vi "KDTHN_Main.vi"() -> ()   [LabVIEW 2018]
doc: "This VIs aim to control both PicoScope 2204A and Arduino UNO3 with ADS9850BRS to gen sinunoid signal with different frequencies\n\nProgrammer: myselfHungNN\n0968354050\nhungtd@mta.edu.vn"
uses:
  LVDrivers_Instruments/uno3/uno3.lvlib
  <vilib>/ErrorRing/Error Ring.xnode
  type defs/TimeBase Cluster.ctl
  type defs/Trigger Cluster.ctl
  type defs/Ranges.ctl
  type defs/Channel Settings.ctl
  type defs/Pico Cluster.ctl
  type defs/Channel Selection.ctl
  LVDrivers_Instruments/picoscope2000a/picoscope2000.lvlib
  type defs/App Cluster.ctl
  type defs/AmplifierTypes.ctl
  type defs/OpAmp Amplifiers.ctl
  <vilib>/Instr/_visa.llb/VISA Configure Serial Port (Instr).vi
panel:
  out "Time left":string
  out "Ngµy & Giê":string
  in  "Test?":bool
  in  "capture":bool caption="L­u mµn h×nh"
  in  "D÷ liÖu  ®o":string[][](table)
  in  "Trans":bool
  in  "OpAmp":bool
  in  "Opamp Type":T1=enum."NO Amplifier" caption="OpAmp"
  in  "Play Button":bool
  in  "Offset":dbl
  in  "Range 2":T2=enum."5 V"
  in  "Coupling":i16(ring)=1 items=["AC", "DC"]
  in  "Enabled":bool=TRUE
  in  "Offset":dbl
  in  "Range":T2=enum."5 V"
  in  "Coupling":i16(ring)=1 items=["AC", "DC"]
  in  "Enabled":bool=TRUE
  in  "Tab Control":enum32{"D¹ng sãng tÝn hiÖu", "Phæ tÝn hiÖu"}(tab)
  out "Time":waveform(dbl)[](graph)
  out "Freq":waveform(dbl)[](graph)
  in  "Disconnect":bool
  in  "Connect":bool
  out "sent":string
  out "number":u8
  out "UNO Rep":string
  in  "# Samples":i32=6000
  in  "Timebase":i16=3
  in  "Direction":i16(ring) items=["Rising", "Falling"]
  in  "Source":i16(ring)=5 items=["Ch A", "Ch B", "Ch C", "Ch D", "Ext", "None"]
  in  "Threshold mV":i16
  out "Actual Sampling Time ns":dbl caption="Actual Sampling Time [ns]"
  out "stop":bool
  in  "Cæng kÕt nèi":refnum<visa-resource-name>="COM4"
  in  "Test Error":bool
  in  "Amplifier Type":T3 caption="Trans Type"
  in  "Amplitude(Volts)":u8(knob)=1 max=10 step=1 scale=0.0..10.0
  in  "Frequency(Hz)":dbl(knob) min=0.0 max=1500000.0 scale=500.0..1500000.0
  in  "Quit Button":bool
  # "M¸Y PH¸T TÝN HIÖU"
  # "M¸Y HIÖN SãNG"
  # "Chan A"
  # "Chan B"
  # "Trigger"
  # "TimeDiv"
  # "khoa v« tuyÕn ®iÖn tö\nBé m«n C¬ së kü thuËt v« tuyÕn"
  # "AMPL"
  # "FREQ"
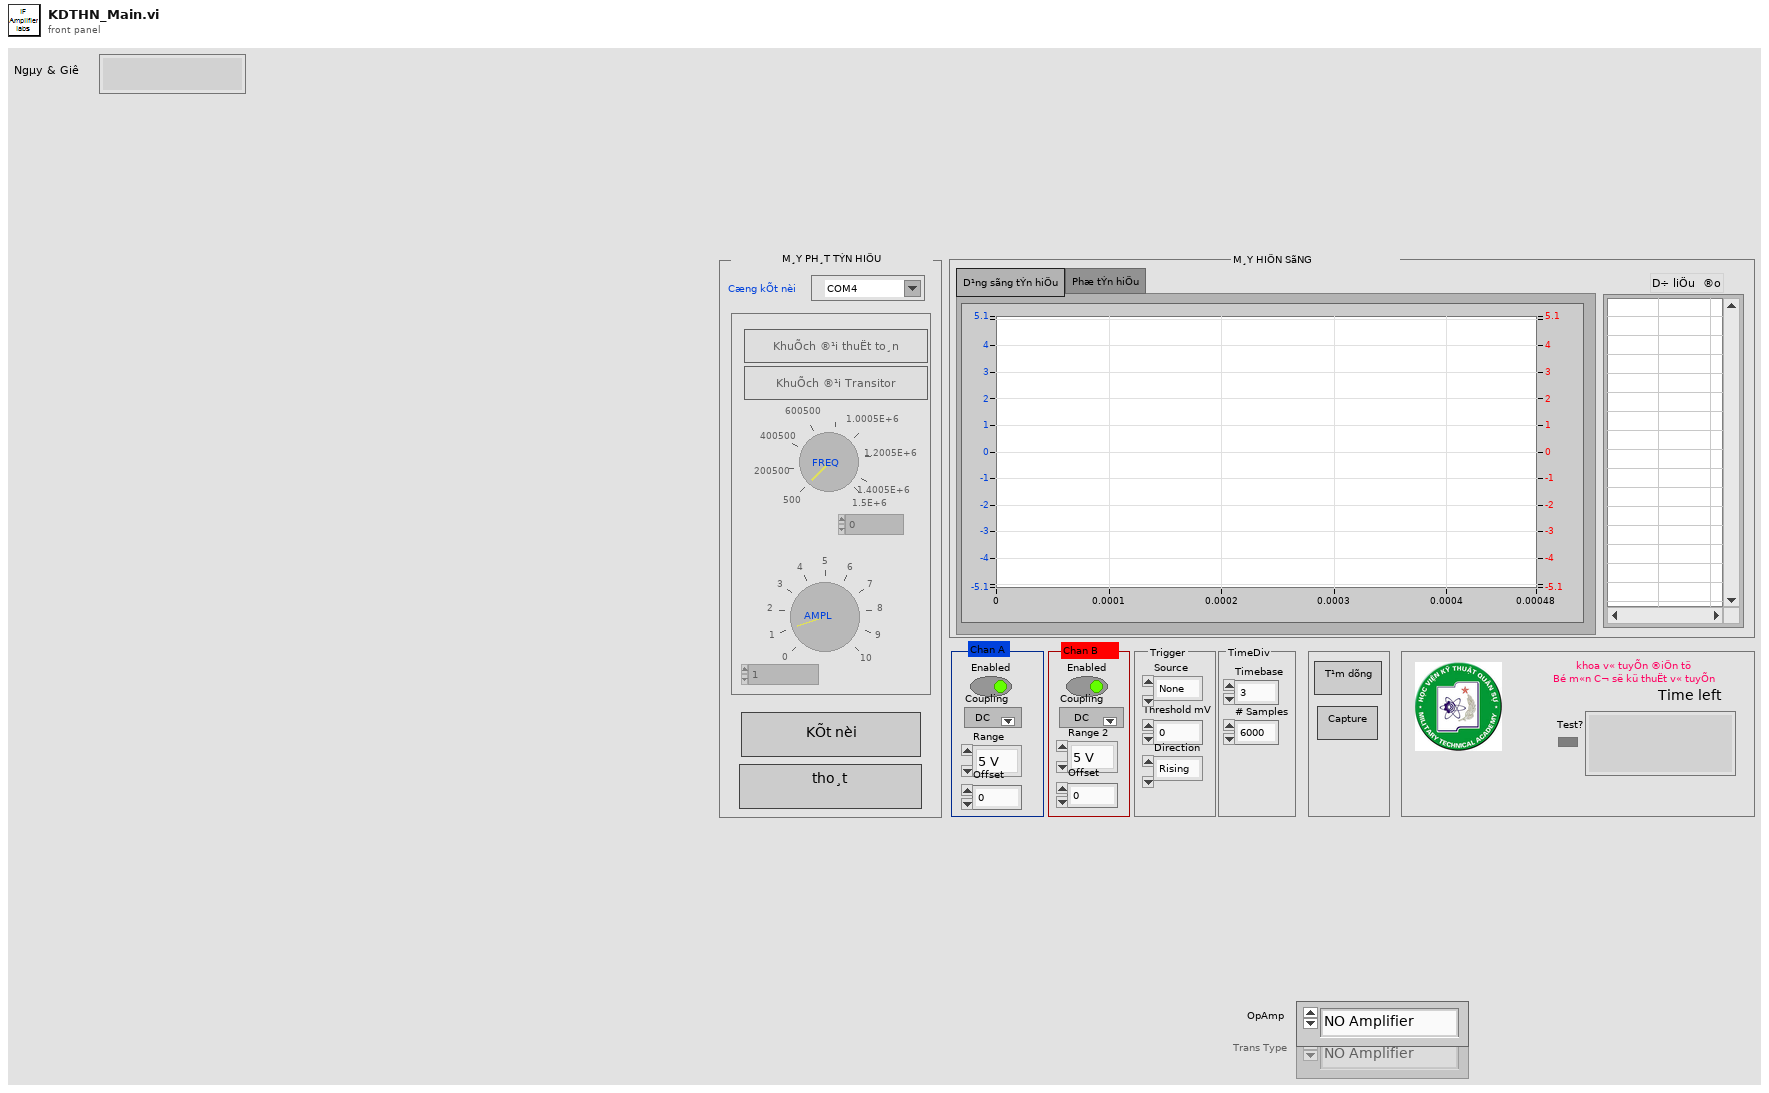
[diagram p1: front panel]
types:
  T1 = typedef "OpAmp Amplifiers.ctl" = enum8{"Inverted Amplifiers", "non-Inverted Amplifiers", "NO Amplifier"}
  T2 = typedef "Ranges.ctl" = enum16{"10 mV", "20 mV", "50 mV", "100 mV", "200 mV", "500 mV", "1 V", "2 V", "5 V", "10 V", "20 V"}
  T3 = typedef "AmplifierTypes.ctl" = enum8{"NO Amplifier", "EC", "BC", "CC"}
  T4 = typedef "Pico Cluster.ctl" = cluster{"Trigger":T5, "TimeBase":T6}
  T5 = typedef "Trigger Cluster.ctl" = cluster{"Direction":i16, "Delay":i16, "Auto Trigger ms":i16, "Threshold mV":i16, "Source":i16}
  T6 = typedef "TimeBase Cluster.ctl" = cluster{"Timebase":i16, "No of samples":i32, "Oversample":i16}
  T7 = typedef "App Cluster.ctl" = cluster{"CMD":string, "Data":variant}
  T8 = enum8{"Enabled", "Disabled", "Disabled and Grayed Out"}
  T9 = typedef "imagedata.ctl" = cluster{"image type":i32, "image depth":i32, "image":u8[], "mask":u8[], "colors":u32[], "Rectangle":cluster{"left":i16, "top":i16, "right":i16, "bottom":i16}}
  T10 = typedef "Channel Settings.ctl" = cluster{"Enabled":bool, "Coupling":i16, "Range":T2, "offset":dbl}
  T11 = typedef "Channel Selection.ctl" = enum16{"channel A", "Channel B", "Channel C", "Channel D", "Ext", "NONE"}
  T12 = typedef "Sampling Infor.ctl" = cluster{"time interval ns":i32, "time_units":i16, "max_sample":i32}
  T13 = typedef "Times&Values.ctl" = cluster{"times":i32[], "bufferA":i16[], "bufferB":i16[]}
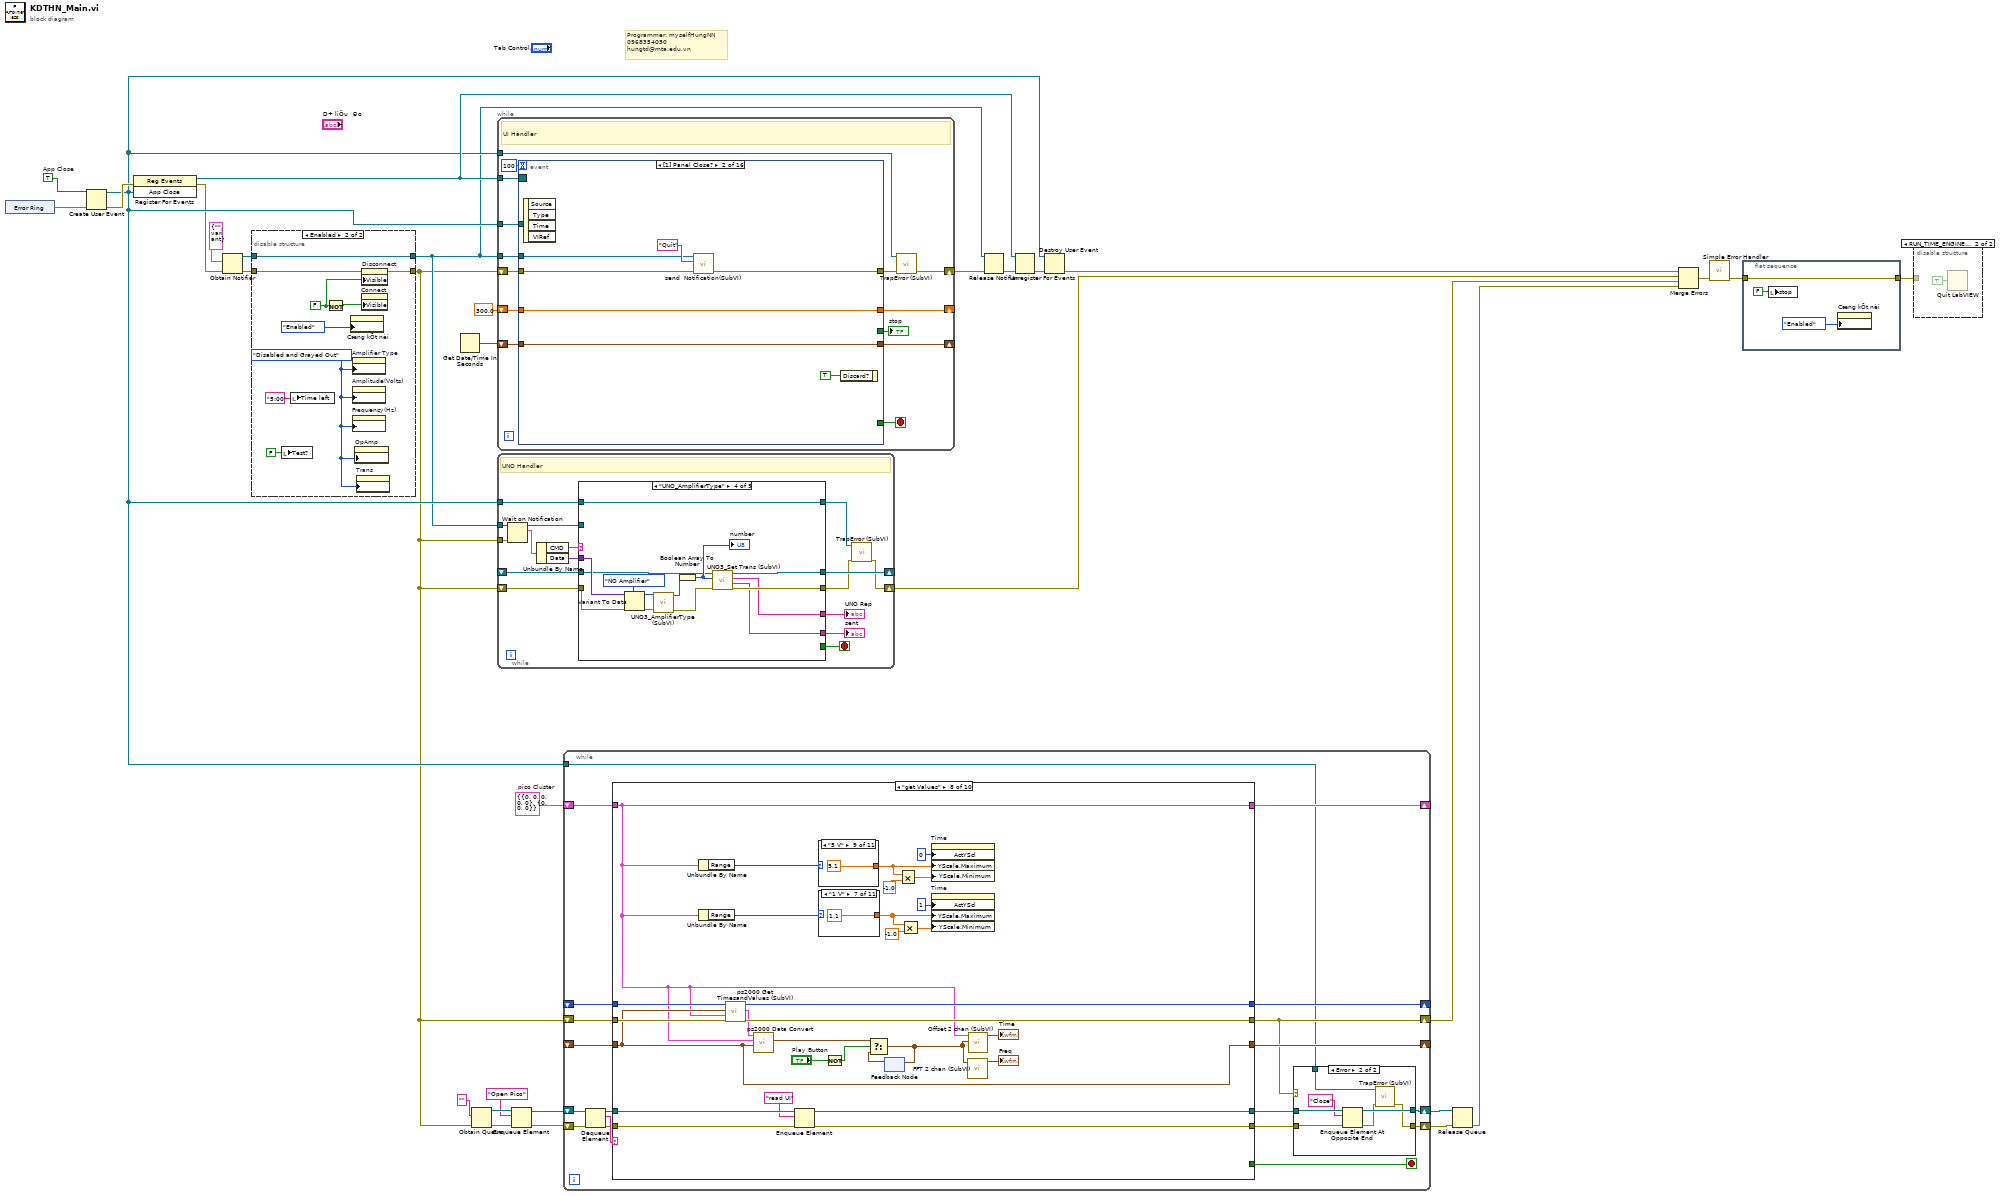
[diagram p0: block diagram]
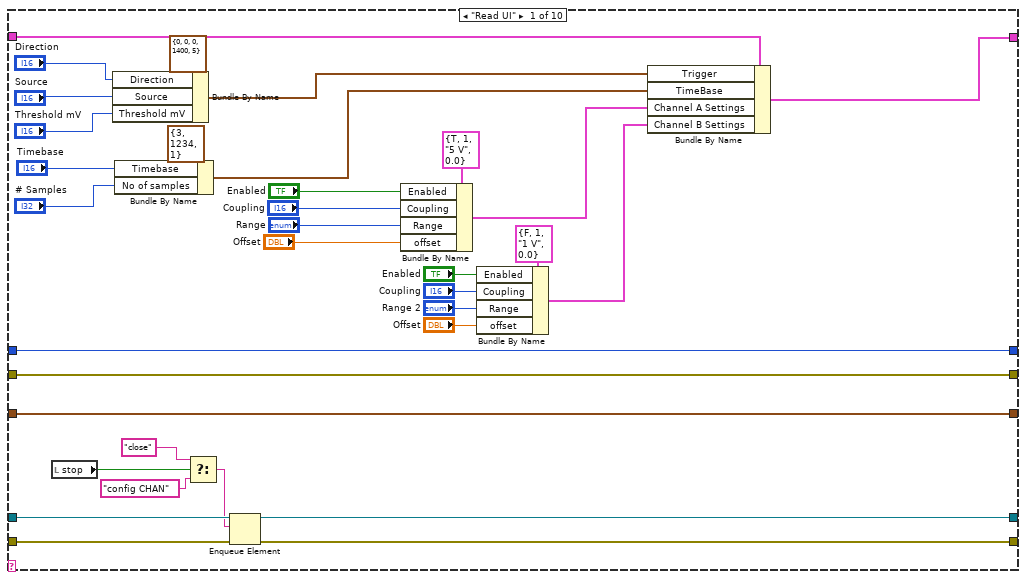
[diagram p3: hidden frame]
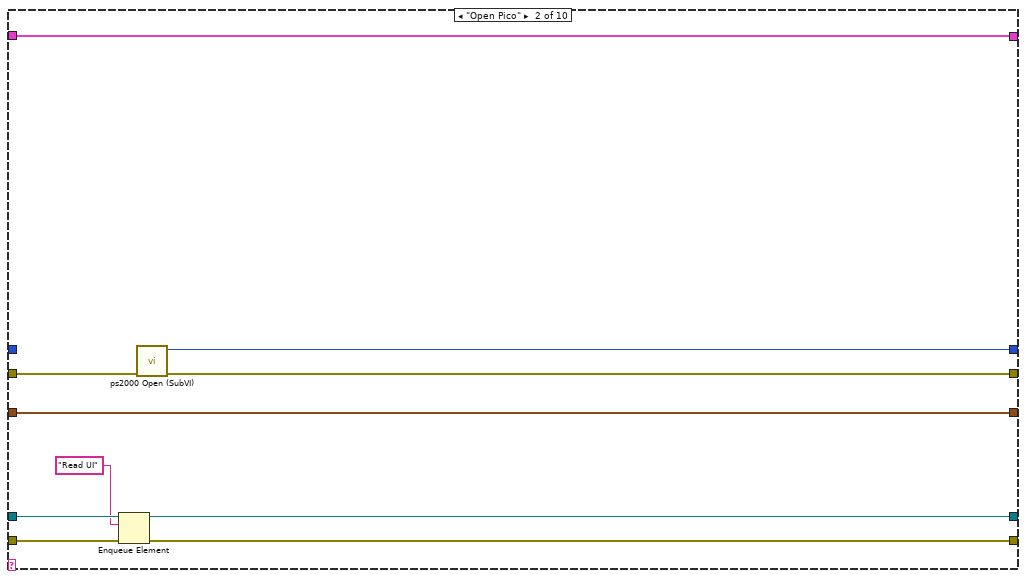
[diagram p4: hidden frame]
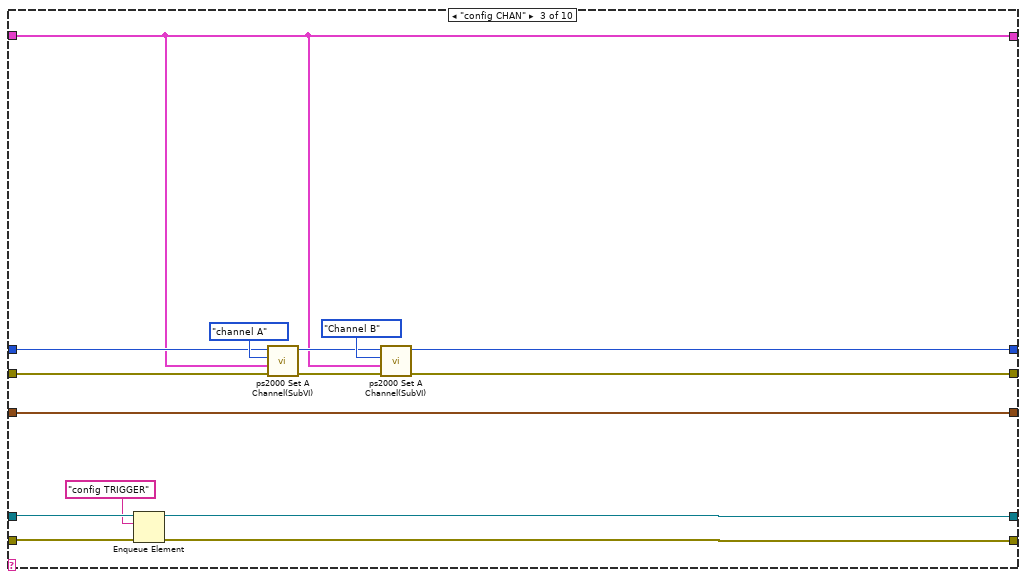
[diagram p5: hidden frame]
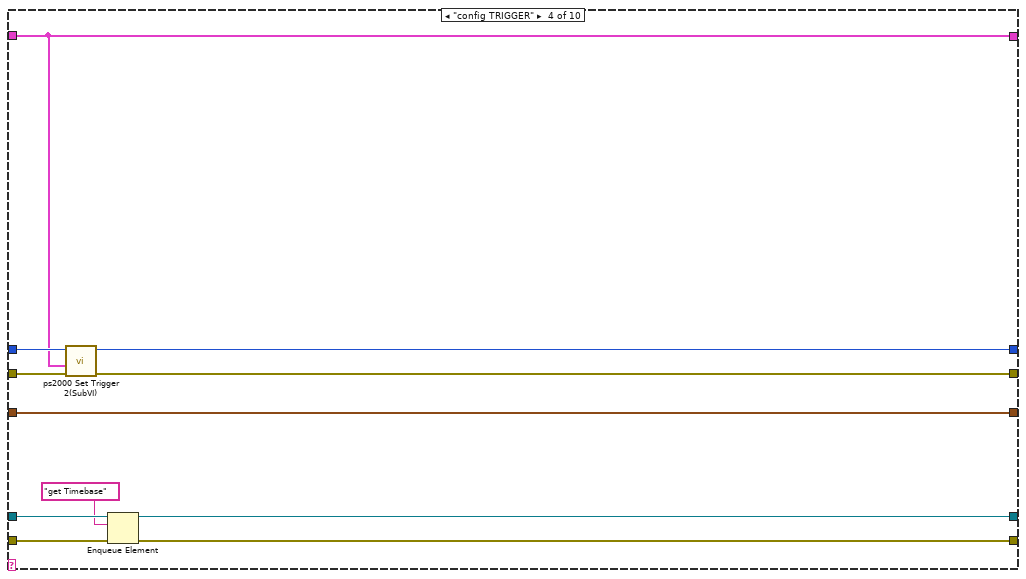
[diagram p6: hidden frame]
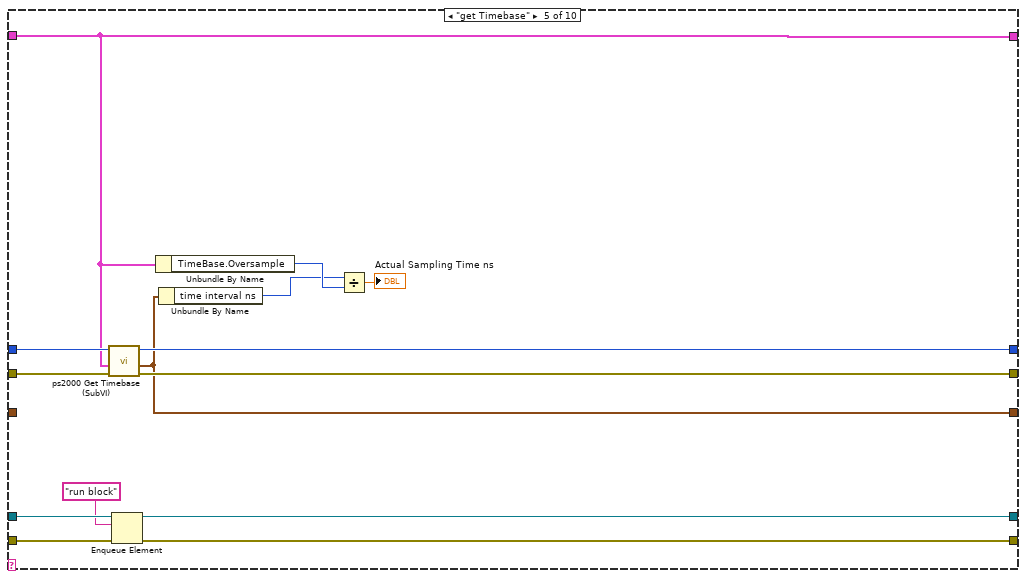
[diagram p7: hidden frame]
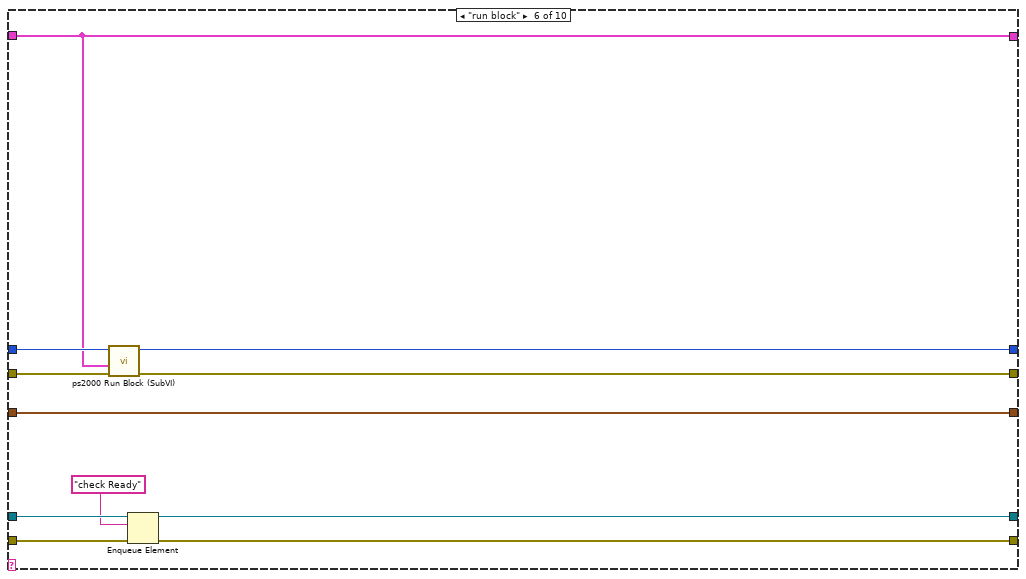
[diagram p8: hidden frame]
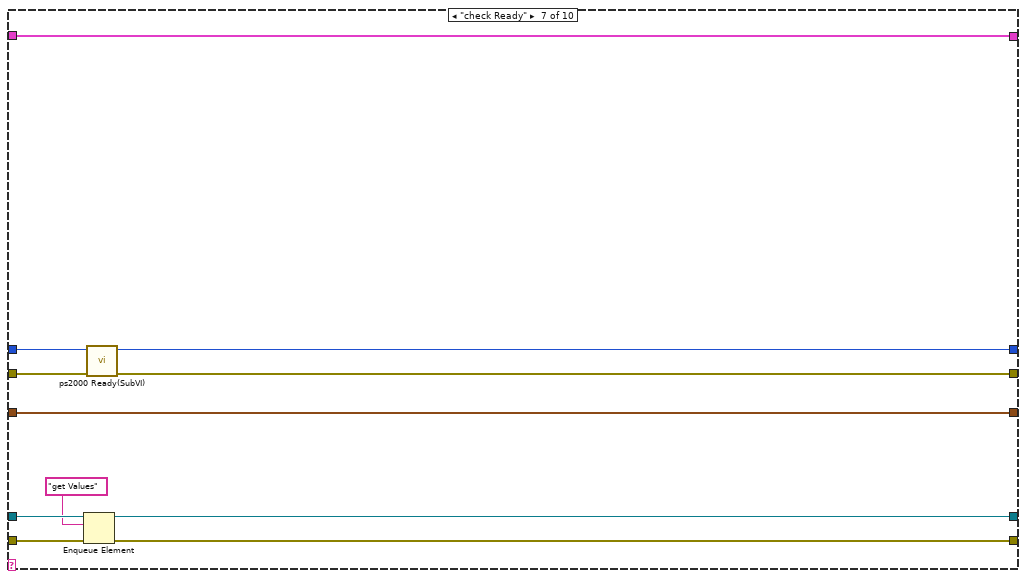
[diagram p9: hidden frame]
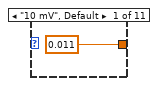
[diagram p10: hidden frame]
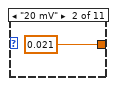
[diagram p11: hidden frame]
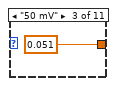
[diagram p12: hidden frame]
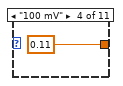
[diagram p13: hidden frame]
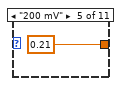
[diagram p14: hidden frame]
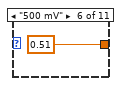
[diagram p15: hidden frame]
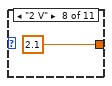
[diagram p16: hidden frame]
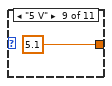
[diagram p17: hidden frame]
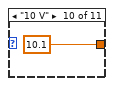
[diagram p18: hidden frame]
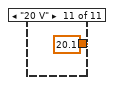
[diagram p19: hidden frame]
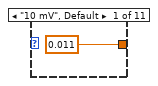
[diagram p20: hidden frame]
diagram:
  w5 = T4 {"Trigger"={"Direction"=0, "Delay"=0, "Auto Trigger ms"=0, "Threshold mV"=0, "Source"=0}, "TimeBase"={"Timebase"=0, "No of samples"=0, "Oversample"=0}}  # pico Cluster
  w32 = TRUE  # App Close
  # "Programmer: myselfHungNN\n0968354050\nhungtd@mta.edu.vn"
  n1 = xnode "Error Ring"() -> ("error out"=w31:errorcluster)
  n2 = Create User Event(user event datatype=w32, error in=w31) -> (user event=w24:refnum<user-event>, error out=w30:errorcluster)
  n3 = register-events(error in=w30, w24) -> (reference out=w29:refnum<event-registration>, error out=w17:errorcluster)  [unwired: 1 in]
  n4 = Obtain Notifier(notification data type=T7 {"CMD"="", "Data"=variant} ("Apps Cluster"), error in (no error)=w17) -> (notifier out=w19:refnum<notifier>, error out=w16:errorcluster)  [unwired: 2 in, 1 out]
  n5 = disable-structure shown="Enabled" {
    disable-tunnel: w19 -> [w37 w46]
    disable-tunnel: [w35 w46] -> w15
    disable-tunnel: w16 -> [w34 w45]
    disable-tunnel: [_ w44] -> w12
    frame Disabled {
      n6 = call "send  Notification(SubVI).vi"("error in (no error)"=w34, "CMD"="INIT", "notifier in"=w37) -> ("error out"=w33:errorcluster, "notifier out"=w35:refnum<notifier>)  [unwired: 7 in]
    }
    frame Enabled {
      w40 = T8."Disabled and Grayed Out" ("Disabled")
      w42 = FALSE ("Visible")
      n7 = local write "Test?"(FALSE ("Test?")) -> ()
      n8 = local write "Time left"("5:00" ("Time left")) -> ()
      n9 = Not(x=w42) -> (.not. x?=w43:bool)
      n10 = property on="Cæng kÕt nèi" class="VISAName"("DisabledEnum"=T8."Enabled" ("Disabled")) -> ()  [unwired: 2 in, 2 out]
      n11 = property on="Amplifier Type" class="Enum (strict)"("DisabledEnum"=w40) -> ()  [unwired: 2 in, 2 out]
      n12 = property on="Amplitude(Volts)" class="Knob (strict)"("DisabledEnum"=w40) -> ()  [unwired: 2 in, 2 out]
      n13 = property on="Frequency(Hz)" class="Knob (strict)"("DisabledEnum"=w40) -> ()  [unwired: 2 in, 2 out]
      n14 = property on="OpAmp" class="Bool"("DisabledEnum"=w40) -> ()  [unwired: 2 in, 2 out]
      n15 = property on="Trans" class="Bool"("DisabledEnum"=w40) -> ()  [unwired: 2 in, 2 out]
      n16 = property on="Disconnect" class="Bool"(error in=w45, "Visible"=w42) -> (error out=w44:errorcluster)  [unwired: 1 in, 1 out]
      n17 = property on="Connect" class="Bool"("Visible"=w43) -> ()  [unwired: 2 in, 2 out]
    }
  }
  n18 = Get Date/Time In Seconds() -> (seconds since 1Jan1904=w1:timestamp)
  n19 = Obtain Queue(element data type="", error in (no error)=w12) -> (queue out=w10:refnum<queue>, error out=w9:errorcluster)  [unwired: 3 in, 1 out]
  n20 = while {
    tunnel: w15 -> [w50]
    tunnel: w12 -> [w47]
    shift-right: [w59] -> _
    shift-left: _ -> [w58]
    shift-right: [w56] -> w25
    shift-left: w12 -> [w57]
    tunnel: w24 -> [w51]
    stop <- w60 stop-if-true
    # "UNO Handler"
    n21 = Wait on Notification(notifier=w50, error in (no error)=w47) -> (notifier out=w49:refnum<notifier>, notification=w48:T7)  [unwired: 2 in, 2 out]
    n22 = Unbundle By Name(w48) -> ("CMD"=w62:string, "Data"=w61:variant)
    n23 = case shown="\"UNO_AmplifierType\"" w62 {
      tunnel: w61 -> [_ _ _ w90 w103 w112 w125 _ _]
      tunnel: [_ TRUE _ _ _ _ _ _ _] -> w60
      tunnel: [w65 _ _ w83 w96 w114 w123 w130 w150] -> w59
      tunnel: w58 -> [w65 w71 w76 w85 w101 w115 w124 w133 _]
      tunnel: [w64 w67 w74 w84 w97 w108 w119 w129 w149] -> w55
      tunnel: w57 -> [w64 w70 w75 w81 w94 w110 w121 w131 w147]
      tunnel: w49 -> [_ _ _ _ _ _ _ _ _]
      tunnel: [_ _ _ w79 w91 w107 w118 w128 _] -> w54
      tunnel: [_ _ _ w78 w95 w106 w117 _ _] -> w53
      tunnel: [w63 w66 w73 w77 w104 w105 w116 w127 w146] -> w52
      tunnel: w51 -> [w63 w66 w73 w77 w104 w105 w116 w127 w146]
      frame "Idle", Default {
      }
      frame "Quit" {
        n24 = VISA Close(VISA resource name=w71, error in (no error)=w70) -> (error out=w68:errorcluster)
        n25 = Generate User Event(user event=w66, event data cluster=TRUE ("event data"), error in=w68) -> (error out=w67:errorcluster)  [unwired: 1 in, 1 out]
      }
      frame "Close COM" {
        n26 = VISA Close(VISA resource name=w76, error in (no error)=w75) -> (error out=w74:errorcluster)
      }
      frame "UNO_AmplifierType" {
        n27 = Variant To Data(error in=w81, type=AmplifierTypes."NO Amplifier" ("Amplifier Type"), Variant=w90) -> (data=w86:T3, error out=w82:errorcluster)
        n28 = call "UNO3_AmplifierType (SubVI).vi"("Error In"=w82, "Amplifier Type"=w86) -> ("Error Out"=w80:errorcluster, "ArrayOut"=w87:bool[])  [unwired: 8 in]
        n29 = Boolean Array To Number(Boolean array=w87) -> (number=w88:u8)
        "number" <- w88
        n30 = call "UNO3_Set Trans (SubVI).vi"("error in (no error)"=w80, "number"=w88, "VISA Refnum in"=w85) -> ("error out"=w84:errorcluster, "Sent"=w78:string, "UNO Rep"=w79:string, "VISA Refnum out"=w83:refnum<visa-resource-name>)  [unwired: 5 in]
      }
      frame "UNO_OpampType" {
        n31 = Variant To Data(error in=w94, type=OpAmp_Amplifiers."Inverted Amplifiers" ("Opamp Type"), Variant=w103) -> (data=w100:T1, error out=w93:errorcluster)
        n32 = call "UNO3_OpampType (SubVI).vi"("Error In"=w93, "Amplifier Type 2"=w100) -> ("Error Out"=w92:errorcluster, "ArrayOut"=w99:bool[])  [unwired: 8 in]
        n33 = Boolean Array To Number(Boolean array=w99) -> (number=w98:u8)
        n34 = call "UNO3_Set Opamps(SubVI).vi"("error in (no error)"=w92, "number"=w98, "VISA Refnum in"=w101) -> ("error out"=w97:errorcluster, "Sent"=w95:string, "UNO Rep"=w91:string, "VISA Refnum out"=w96:refnum<visa-resource-name>)  [unwired: 5 in]
      }
      frame "Amplitude(Volts)" {
        n35 = Variant To Data(error in=w110, type=u8 0 ("Amplitude(Volts)"), Variant=w112) -> (data=w111:u8, error out=w109:errorcluster)
        n36 = call "UNO3 Set Amplitude (SubVI).vi"("error in (no error)"=w109, "Amplitude"=w111, "VISA Refnum in"=w115) -> ("error out"=w108:errorcluster, "sent"=w106:string, "UNO Rep"=w107:string, "VISA Refnum out"=w114:refnum<visa-resource-name>)  [unwired: 5 in]
      }
      frame "Frequency(Hz)" {
        n37 = Variant To Data(error in=w121, type=0.0 ("Frequency(Hz)"), Variant=w125) -> (data=w122:dbl, error out=w120:errorcluster)
        n38 = call "ads9850_setFreq (SubVI).vi"("error in (no error)"=w120, "Frequency(Hz)"=w122, "VISA Refnum in"=w124) -> ("error out"=w119:errorcluster, "concatenated string"=w117:string, "UNO rep"=w118:string, "VISA Refnum out"=w123:refnum<visa-resource-name>)  [unwired: 5 in]
      }
      frame "UNO_Read" {
        n39 = flat-sequence {
          tunnel: [w136] -> w134
          tunnel: w133 -> [w136]
          tunnel: [w135] -> w132
          tunnel: w131 -> [w135]
          tunnel: w134 -> [w145]
          tunnel: w132 -> [w144]
          tunnel: [w140] -> w130
          tunnel: [w139] -> w129
          tunnel: [w138] -> w128
          frame #0 {
            n40 = Wait (ms)(milliseconds to wait=u32 100) -> ()  [unwired: 1 out]
          }
          frame #1 {
            n41 = property class="Instr"(reference=w145, error in=w144) -> (reference out=w143:refnum<visa-resource-name>, error out=w142:errorcluster, "Serial Settings:Number of Bytes at Serial Port"=w141:u32)
            n42 = VISA Read(VISA resource name=w143, byte count=w141, error in (no error)=w142) -> (VISA resource name out=w140:refnum<visa-resource-name>, read buffer=w138:string, error out=w139:errorcluster)  [unwired: 1 out]
          }
        }
      }
      frame "Open COM" {
        n43 = call-poly "VISA Configure Serial Port"("VISA resource name"="Cæng kÕt nèi", "error in (no error)"=w147) -> ("VISA resource name out"=w150:refnum<visa-resource-name>, "error out"=w149:errorcluster)  [unwired: 12 in]
      }
    }
    "UNO Rep" <- w54
    "sent" <- w53
    n44 = call "TrapError (SubVI).vi"("error in (no error)"=w55, "stopEvent in"=w52) -> ("error out"=w56:errorcluster)  [unwired: 8 in, 1 out]
  }
  n45 = while {
    shift-right: [w161] -> w14
    shift-left: w12 -> [w160]
    tunnel: w29 -> [w164]
    tunnel: w15 -> [w158]
    tunnel: w24 -> [w159]
    tunnel: w24 -> [w157]
    shift-right: [w154] -> _
    shift-left: 300.0 ("Test Duration(min)") -> [w153]
    shift-right: [w152] -> _
    shift-left: w1 -> [w151]
    stop <- w163 stop-if-true
    # "UI Handler"
    n46 = event shown="[1] Panel Close?" {
      selector: w164 -> [_ _ _ _ _ _ _ _ _ _ _ _ _ _ _ _]
      dyn-events: _ -> [_ _ _ _ _ _ _ _ _ _ _ _ _ _ _ _]
      timeout: 100 -> [_ _ _ _ _ _ _ _ _ _ _ _ _ _ _ _]
      tunnel: w158 -> [w170 w176 w183 w197 _ w240 w253 _ w285 w298 _ w313 _ w328 w338 _]
      tunnel: [w167 w174 w181 w195 _ w237 w244 w263 w290 w296 w304 w309 w317 w326 w333 w347] -> w162
      tunnel: w160 -> [w168 w175 w182 w196 _ w239 w252 w263 w286 w297 w306 w310 w320 w327 w337 w349]
      tunnel: [w171 _ _ _ _ _ _ _ _ _ _ _ _ _ _ _] -> w163
      tunnel: w157 -> [_ _ _ _ _ _ _ _ _ _ _ _ _ _ _ _]
      tunnel: [w171 _ _ _ _ _ _ _ _ _ _ _ _ _ _ _] -> w156
      tunnel: w153 -> [w166 w173 w180 w188 _ w236 w242 w256 w284 w294 w302 w308 w316 w322 w330 w344]
      tunnel: [w166 w173 w180 w188 w227 w236 w242 w256 w284 w294 w302 w308 w316 w322 w330 w344] -> w154
      tunnel: [w165 w172 w179 w186 w226 w235 w241 w255 w283 w293 w301 w307 w315 w321 w329 w343] -> w152
      tunnel: w151 -> [w165 w172 w179 w186 _ w235 w241 w255 w283 w293 w301 w307 w315 w321 w329 w343]
      event User Event {
        w171 = TRUE
        n47 = event-data() -> ()  [unwired: 1 in, 5 out]
        n48 = call "send  Notification(SubVI).vi"("error in (no error)"=w168, "CMD"="Quit", "notifier in"=w170) -> ("error out"=w167:errorcluster)  [unwired: 7 in, 1 out]
      }
      event Panel Close? {
        n49 = event-data() -> ()  [unwired: 1 in, 4 out]
        n50 = call "send  Notification(SubVI).vi"("error in (no error)"=w175, "CMD"="Quit", "notifier in"=w176) -> ("error out"=w174:errorcluster)  [unwired: 7 in, 1 out]
        n51 = event-data("Discard?"=TRUE) -> ()  [unwired: 1 in, 1 out]
      }
      event Menu Selection? (App) {
        n52 = event-data() -> ()  [unwired: 1 in, 3 out]
        n53 = call "send  Notification(SubVI).vi"("error in (no error)"=w182, "CMD"="Quit", "notifier in"=w183) -> ("error out"=w181:errorcluster)  [unwired: 7 in, 1 out]
        n54 = event-data("Discard?"=TRUE) -> ()  [unwired: 1 in, 1 out]
      }
      event Timeout {
        n55 = event-data() -> ()  [unwired: 1 in, 3 out]
        n56 = local read "Test?"() -> (w189:bool)
        n57 = Get Date/Time String(date format (0)=enum16{"short", "long", "abbreviated"}."short") -> (date string=w192:string, time string=w193:string)  [unwired: 2 in]
        n58 = case shown="True" w189 {
          tunnel: w186 -> [_ w217]
          tunnel: w188 -> [_ w214]
          tunnel: [_ w212] -> w187
          frame False {
          }
          frame True {
            n59 = Get Date/Time In Seconds() -> (seconds since 1Jan1904=w215:timestamp)
            n60 = Subtract(x=w215, y=w217) -> (x-y=w216:dbl)
            n61 = Round To Nearest(number=w216) -> (nearest integer value=w213:dbl)
            n62 = Subtract(x=w214, y=w213) -> (x-y=w211:dbl)
            n63 = Quotient & Remainder(x=w211, y=60.0) -> (x-y*floor(x/y)=w208:dbl, floor(x/y)=w209:dbl)
            n64 = Less Or Equal To 0?(x=w211) -> (x <= 0?=w212:bool)
            n65 = Number To Decimal String(number=w208) -> (decimal integer string=w199:string)  [unwired: 1 in]
            n66 = Number To Decimal String(number=w209) -> (decimal integer string=w207:string)  [unwired: 1 in]
            n67 = String Length(string=w199) -> (length=w203:i32)
            n68 = Concatenate Strings("0" ("string"), w199) -> (w200:string)
            n69 = Less?(x=w203, y=2) -> (x < y?=w201:bool)
            n70 = Select(t=w200, s=w201, f=w199) -> (s? t:f=w198:string)
            n71 = Concatenate Strings(w207, ":" ("string"), w198) -> (→"Time left":string)
          }
        }
        n72 = call <vilib>:"Space Constant.vi"() -> ("String"=w191:string)
        n73 = Concatenate Strings(w192, w191, w193) -> (→"Ngµy & Giê":string)
        n74 = case shown="True" w187 {
          tunnel: w197 -> [_ w224]
          tunnel: w196 -> [w218 w223]
          tunnel: [w218 w222] -> w195
          frame False {
          }
          frame True {
            n75 = call "send  Notification(SubVI).vi"("error in (no error)"=w223, "CMD"="Quit", "notifier in"=w224) -> ("error out"=w222:errorcluster)  [unwired: 7 in, 1 out]
            n76 = call <vilib>:"Beep.vi"("duration (msec)"=u32 2000) -> ()  [unwired: 11 in]
            n77 = One Button Dialog(message="Time Out!!!!!!!", button name ("OK")="OK") -> ()  [unwired: 1 out]
          }
        }
      }
      event "Test?": Value Change {
        n78 = event-data() -> ("NewVal"=w228:bool)  [unwired: 1 in, 5 out]
        n79 = case shown="True" w228 {
          tunnel: [_ w230] -> w227
          tunnel: [_ w232] -> w226
          frame False {
          }
          frame True {
            n80 = call "Read TestDuration.vi"() -> ("Test Duration(min)"=w234:dbl)  [unwired: 10 in, 1 out]
            n81 = Get Date/Time In Seconds() -> (seconds since 1Jan1904=w232:timestamp)
            n82 = local write "Time left"("5:00" ("Time left")) -> ()
            n83 = Multiply(x=w234, y=60.0) -> (x*y=w231:dbl)
            n84 = Round To Nearest(number=w231) -> (nearest integer value=w230:dbl)
          }
        }
      }
      event "Quit Button": Value Change {
        n85 = event-data() -> ()  [unwired: 1 in, 2 out]
        n86 = call "send  Notification(SubVI).vi"("error in (no error)"=w239, "CMD"="Quit", "notifier in"=w240) -> ("error out"=w237:errorcluster)  [unwired: 7 in, 1 out]
      }
      event "Connect": Value Change {
        w247 = T8."Enabled" ("Disabled")
        w249 = FALSE ("Visible")
        n87 = event-data() -> ()  [unwired: 1 in, 1 out]
        n88 = Not(x=w249) -> (.not. x?=w250:bool)
        n89 = property on="Connect" class="Bool"("Visible"=w249) -> ()  [unwired: 2 in, 2 out]
        n90 = property on="Disconnect" class="Bool"("Visible"=w250) -> ()  [unwired: 2 in, 2 out]
        n91 = call "send  Notification(SubVI).vi"("error in (no error)"=w252, "CMD"="Open COM", "notifier in"=w253) -> ("error out"=w251:errorcluster)  [unwired: 7 in, 1 out]
        n92 = property on="Frequency(Hz)" class="Knob (strict)"(error in=w251, "Val(Sgnl)"=100000.0 ("Value (Signaling)")) -> (error out=w245:errorcluster)  [unwired: 1 in, 1 out]
        n93 = property on="Cæng kÕt nèi" class="VISAName"("DisabledEnum"=T8."Disabled and Grayed Out" ("Disabled")) -> ()  [unwired: 2 in, 2 out]
        n94 = property on="Amplitude(Volts)" class="Knob (strict)"(error in=w245, "Val(Sgnl)"=u8 4 ("Value (Signaling)")) -> (error out=w244:errorcluster)  [unwired: 1 in, 1 out]
        n95 = property on="Amplifier Type" class="Enum (strict)"("DisabledEnum"=w247) -> ()  [unwired: 2 in, 2 out]
        n96 = property on="Amplitude(Volts)" class="Knob (strict)"("DisabledEnum"=w247) -> ()  [unwired: 2 in, 2 out]
        n97 = property on="Frequency(Hz)" class="Knob (strict)"("DisabledEnum"=w247) -> ()  [unwired: 2 in, 2 out]
        n98 = property on="OpAmp" class="Bool"("DisabledEnum"=w247) -> ()  [unwired: 2 in, 2 out]
        n99 = property on="Trans" class="Bool"("DisabledEnum"=w247) -> ()  [unwired: 2 in, 2 out]
      }
      event "capture": Value Change {
        n100 = event-data() -> ()  [unwired: 1 in, 6 out]
        n101 = control-ref of="This VI"() -> (w262:refnum<vi>)
        n102 = invoke class="VI" method="FP.Get Image"(reference=w262) -> ("image data"=w261:T9)  [unwired: 5 in, 5 out]
        n103 = First Call?() -> (First Call?: T/F=w260:bool)
        n104 = feedback #1() -> (w259:path)  [unwired: 1 in]
        n105 = case shown="False" w260 {
          tunnel: [w273 w279] -> w257
          tunnel: w259 -> [w264 _]
          tunnel: [w264 w279] -> w258
          frame False {
            n106 = Path To String(path=w264) -> (string=w270:string)
            n107 = String Length(string=w270) -> (length=w269:i32)
            n108 = Subtract(x=w269, y=4) -> (x-y=w267:i32)
            n109 = Subtract(x=w269, y=4) -> (x-y=w271:i32)
            n110 = String Subset(string=w270, length (rest)=w267) -> (substring=w266:string)  [unwired: 1 in]
            n111 = String Subset(string=w270, offset (0)=w271) -> (substring=w265:string)  [unwired: 1 in]
            n112 = feedback #2(0) -> (w275:i32)
            n113 = Number To Decimal String(number=w275) -> (decimal integer string=w278:string)  [unwired: 1 in]
            n114 = Concatenate Strings(w266, w278, w265) -> (w274:string)
            n115 = Increment(x=w275) -> (x+1=w277:i32)
            n116 = feedback-in #2(w277) -> ()
            n117 = String To Path(string=w274) -> (path=w273:path)
          }
          frame True {
            n118 = call "File Dialog"("start path"=path "C:/Users/HP/Desktop", "pattern (all files)"="*.jpg", "pattern label"="") -> ("selected path"=w279:path)  [unwired: 9 in, 3 out]
          }
        }
        n119 = feedback-in #1(w258) -> ()
        n120 = call <vilib>:"Write JPEG File.vi"("image data"=w261, "path to JPEG file"=w257) -> ()  [unwired: 8 in, 2 out]
      }
      event "Disconnect": Value Change {
        w287 = T8."Disabled and Grayed Out" ("Disabled")
        w291 = TRUE ("Visible")
        n121 = event-data() -> ()  [unwired: 1 in, 6 out]
        n122 = property on="Cæng kÕt nèi" class="VISAName"("DisabledEnum"=T8."Enabled" ("Disabled")) -> ()  [unwired: 2 in, 2 out]
        n123 = Not(x=w291) -> (.not. x?=w292:bool)
        n124 = property on="Connect" class="Bool"("Visible"=w291) -> ()  [unwired: 2 in, 2 out]
        n125 = property on="Disconnect" class="Bool"("Visible"=w292) -> ()  [unwired: 2 in, 2 out]
        n126 = property on="Amplifier Type" class="Enum (strict)"("DisabledEnum"=w287) -> ()  [unwired: 2 in, 2 out]
        n127 = property on="Amplitude(Volts)" class="Knob (strict)"("DisabledEnum"=w287) -> ()  [unwired: 2 in, 2 out]
        n128 = property on="Frequency(Hz)" class="Knob (strict)"("DisabledEnum"=w287) -> ()  [unwired: 2 in, 2 out]
        n129 = property on="OpAmp" class="Bool"("DisabledEnum"=w287) -> ()  [unwired: 2 in, 2 out]
        n130 = property on="Trans" class="Bool"("DisabledEnum"=w287) -> ()  [unwired: 2 in, 2 out]
        n131 = call "send  Notification(SubVI).vi"("error in (no error)"=w286, "CMD"="Close COM", "notifier in"=w285) -> ("error out"=w290:errorcluster)  [unwired: 7 in, 1 out]
      }
      event Value Change {
        n132 = event-data() -> ()  [unwired: 1 in, 2 out]
        n133 = To Variant(anything="Amplifier Type") -> (Variant=w299:variant)
        n134 = call "send  Notification(SubVI).vi"("error in (no error)"=w297, "Variant"=w299, "CMD"="UNO_AmplifierType", "notifier in"=w298) -> ("error out"=w296:errorcluster)  [unwired: 6 in, 1 out]
      }
      event "Trans": Value Change {
        n135 = event-data() -> ()  [unwired: 1 in, 6 out]
        n136 = call "Select Trans.vi"("error in (no error)"=w306) -> ("error out"=w305:errorcluster, "Amplifier Type 2"=w303:T3)  [unwired: 9 in]
        n137 = property on="Amplifier Type" class="Enum (strict)"(error in=w305, "Val(Sgnl)"=w303) -> (error out=w304:errorcluster)  [unwired: 1 in, 1 out]
      }
      event Value Change {
        n138 = event-data() -> ()  [unwired: 1 in, 1 out]
        n139 = To Variant(anything="Opamp Type") -> (Variant=w311:variant)
        n140 = call "send  Notification(SubVI).vi"("error in (no error)"=w310, "Variant"=w311, "CMD"="UNO_OpampType", "notifier in"=w313) -> ("error out"=w309:errorcluster)  [unwired: 6 in, 1 out]
      }
      event "OpAmp": Value Change {
        n141 = event-data() -> ()  [unwired: 1 in, 6 out]
        n142 = call "Select Opamp.vi"("error in (no error)"=w320) -> ("error out"=w318:errorcluster, "Opamp Type"=w319:T1)  [unwired: 9 in]
        n143 = property on="Opamp Type" class="Enum (strict)"(error in=w318, "Val(Sgnl)"=w319) -> (error out=w317:errorcluster)  [unwired: 1 in, 1 out]
      }
      event "Amplitude(Volts)": Value Change {
        n144 = event-data() -> ()  [unwired: 1 in, 2 out]
        n145 = To Variant(anything="Amplitude(Volts)") -> (Variant=w323:variant)
        n146 = call "send  Notification(SubVI).vi"("error in (no error)"=w327, "Variant"=w323, "CMD"="Amplitude(Volts)", "notifier in"=w328) -> ("error out"=w326:errorcluster)  [unwired: 6 in, 1 out]
      }
      event "Frequency(Hz)": Value Change {
        n147 = event-data() -> ()  [unwired: 1 in, 3 out]
        n148 = To Variant(anything="Frequency(Hz)") -> (Variant=w331:variant)
        n149 = call "send  Notification(SubVI).vi"("error in (no error)"=w337, "Variant"=w331, "CMD"="Frequency(Hz)", "notifier in"=w338) -> ("error out"=w334:errorcluster)  [unwired: 6 in, 1 out]
        n150 = First Call?() -> (First Call?: T/F=w335:bool)
        n151 = case shown="True" w335 {
          tunnel: w334 -> [w339 w342]
          tunnel: [w339 w341] -> w333
          frame False {
          }
          frame True {
            n152 = property on="Amplifier Type" class="Enum (strict)"(error in=w342, "Val(Sgnl)"=AmplifierTypes."NO Amplifier" ("Value (Signaling)")) -> (error out=w341:errorcluster)  [unwired: 1 in, 1 out]
          }
        }
      }
      event "Test Error": Value Change {
        n153 = event-data() -> ()  [unwired: 1 in, 1 out]
        n154 = Bundle By Name(cluster=w349, "status"=TRUE, "code"=-8000, "source"="User Gen Error") -> (w347:errorcluster)
      }
    }
    "stop" <- w156
    n155 = call "TrapError (SubVI).vi"("error in (no error)"=w162, "stopEvent in"=w159) -> ("error out"=w161:errorcluster)  [unwired: 8 in, 1 out]
  }
  n156 = Enqueue Element(queue=w10, element="Open Pico", error in (no error)=w9) -> (queue out=w7:refnum<queue>, error out=w8:errorcluster)  [unwired: 1 in, 1 out]
  n157 = while {
    shift-right: [w352] -> w4
    shift-left: w7 -> [w368]
    shift-right: [w351] -> w3
    shift-left: w8 -> [w366]
    shift-right: [w364] -> _
    shift-left: w5 -> [w365]
    shift-right: [w361] -> _
    shift-left: _ -> [w360]
    shift-right: [w355] -> w22
    shift-left: w12 -> [w359]
    shift-right: [w358] -> _
    shift-left: _ -> [w357]
    tunnel: w24 -> [w350]
    stop <- w356 stop-if-true
    n158 = Dequeue Element(queue=w368, error in (no error)=w366) -> (queue out=w363:refnum<queue>, element=w367:string, error out=w362:errorcluster)  [unwired: 1 in, 1 out]
    n159 = case shown="\"get Values\"" w367 {
      tunnel: w365 -> [w411 w421 w429 w443 w451 w468 w474 w497 w535 w549]
      tunnel: [w410 w421 w429 w443 w451 w468 w474 w497 w535 w549] -> w364
      tunnel: w363 -> [w409 w420 w426 w442 w460 w466 w479 w504 w538 w545]
      tunnel: w362 -> [w408 w419 w427 w441 w461 w467 w478 w506 w537 w544]
      tunnel: [w407 w417 w424 w439 w458 w464 w476 w503 w538 w545] -> w354
      tunnel: [w406 w418 w425 w440 w459 w465 w477 w505 w537 w544] -> w353
      tunnel: [w405 w412 w432 w444 w454 w469 w480 w510 i16 0 ("handle") w548] -> w361
      tunnel: w360 -> [w405 _ w433 w446 w456 w472 w481 w512 w541 w548]
      tunnel: [w404 w414 w431 w445 w455 w470 w482 w509 w542 w547] -> w355
      tunnel: w359 -> [w404 w413 w428 w447 w457 w471 w483 w511 w543 w547]
      tunnel: [w403 w415 w422 w437 w452 w462 w473 w507 w539 w546] -> w358
      tunnel: w357 -> [w403 w415 w422 w437 _ w462 w473 w507 w539 w546]
      tunnel: [_ _ _ _ _ _ _ _ TRUE _] -> w356
      frame "Read UI" {
        n160 = local read "stop"() -> (w399:bool)
        n161 = Bundle By Name(cluster=T5 {"Direction"=0, "Delay"=0, "Auto Trigger ms"=0, "Threshold mV"=1400, "Source"=5} ("Trigger"), "Direction"="Direction", "Source"="Source", "Threshold mV"="Threshold mV") -> (w396:T5)
        n162 = Bundle By Name(cluster=T6 {"Timebase"=3, "No of samples"=1234, "Oversample"=1} ("TimeBase"), "Timebase"="Timebase", "No of samples"="# Samples") -> (w392:T6)
        n163 = Select(t="close", s=w399, f="config CHAN" ("element")) -> (s? t:f=w401:string)
        n164 = Enqueue Element(queue=w409, element=w401, error in (no error)=w408) -> (queue out=w407:refnum<queue>, error out=w406:errorcluster)  [unwired: 1 in, 1 out]
        n165 = Bundle By Name(cluster=T10 {"Enabled"=TRUE, "Coupling"=1, "Range"=enum."5 V", "offset"=0.0} ("Channel A Settings"), "Enabled"="Enabled", "Coupling"="Coupling", "Range"="Range", "offset"="Offset") -> (w384:T10)
        n166 = Bundle By Name(cluster=T10 {"Enabled"=FALSE, "Coupling"=1, "Range"=enum."1 V", "offset"=0.0} ("Channel B Settings"), "Enabled"="Enabled", "Coupling"="Coupling", "Range"="Range 2", "offset"="Offset") -> (w378:T10)
        n167 = Bundle By Name(cluster=w411, "Trigger"=w396, "TimeBase"=w392, "Channel A Settings"=w384, "Channel B Settings"=w378) -> (w410:T4)
      }
      frame "Open Pico" {
        n168 = Enqueue Element(queue=w420, element="Read UI", error in (no error)=w419) -> (queue out=w417:refnum<queue>, error out=w418:errorcluster)  [unwired: 1 in, 1 out]
        n169 = call "ps2000 Open (SubVI).vi"("error in (no error)"=w413) -> ("error out"=w414:errorcluster, "handle"=w412:i16)  [unwired: 9 in]
      }
      frame "config CHAN" {
        n170 = Enqueue Element(queue=w426, element="config TRIGGER", error in (no error)=w427) -> (queue out=w424:refnum<queue>, error out=w425:errorcluster)  [unwired: 1 in, 1 out]
        n171 = call "ps2000 Set A Channel(SubVI).vi"("error in (no error)"=w428, "pico Cluster"=w429, "Channel"=Channel_Selection."channel A", "handle in"=w433) -> ("error out"=w430:errorcluster, "handle out"=w435:i16)  [unwired: 5 in, 1 out]
        n172 = call "ps2000 Set A Channel(SubVI).vi"("error in (no error)"=w430, "pico Cluster"=w429, "Channel"=Channel_Selection."Channel B", "handle in"=w435) -> ("error out"=w431:errorcluster, "handle out"=w432:i16)  [unwired: 5 in, 1 out]
      }
      frame "config TRIGGER" {
        n173 = call "ps2000 Set Trigger 2(SubVI).vi"("error in (no error)"=w447, "pico Cluster"=w443, "Handle"=w446) -> ("error out"=w445:errorcluster, "handle"=w444:i16)  [unwired: 7 in]
        n174 = Enqueue Element(queue=w442, element="get Timebase", error in (no error)=w441) -> (queue out=w439:refnum<queue>, error out=w440:errorcluster)  [unwired: 1 in, 1 out]
      }
      frame "get Timebase" {
        n175 = call "ps2000 Get Timebase (SubVI).vi"("error in (no error)"=w457, "pico Cluster"=w451, "handle in"=w456) -> ("error out"=w455:errorcluster, "Sampling infor"=w452:T12, "handle out"=w454:i16)  [unwired: 5 in, 1 out]
        n176 = Enqueue Element(queue=w460, element="run block", error in (no error)=w461) -> (queue out=w458:refnum<queue>, error out=w459:errorcluster)  [unwired: 1 in, 1 out]
        n177 = Unbundle By Name(w451) -> ("TimeBase.Oversample"=w450:i16)
        n178 = Unbundle By Name(w452) -> ("time interval ns"=w449:i32)
        n179 = Divide(x=w449, y=w450) -> (x/y=→"Actual Sampling Time ns":dbl)
      }
      frame "run block" {
        n180 = call "ps2000 Run Block (SubVI).vi"("error in (no error)"=w471, "pico Cluster"=w468, "handle in"=w472) -> ("error out"=w470:errorcluster, "handle out"=w469:i16)  [unwired: 5 in, 2 out]
        n181 = Enqueue Element(queue=w466, element="check Ready", error in (no error)=w467) -> (queue out=w464:refnum<queue>, error out=w465:errorcluster)  [unwired: 1 in, 1 out]
      }
      frame "check Ready" {
        n182 = Enqueue Element(queue=w479, element="get Values", error in (no error)=w478) -> (queue out=w476:refnum<queue>, error out=w477:errorcluster)  [unwired: 1 in, 1 out]
        n183 = call "ps2000 Ready(SubVI).vi"("error in (no error)"=w483, "handle in"=w481) -> ("error out"=w482:errorcluster, "handle out"=w480:i16)  [unwired: 7 in, 1 out]
      }
      frame "get Values" {
        n184 = Unbundle By Name(w497) -> ("Range"=w501:T2)
        n185 = Unbundle By Name(w497) -> ("Range"=w496:T2)
        n186 = call "ps2000 Get TimesandValues (SubVI).vi"("error in (no error)"=w511, "pico Cluster"=w497, "Sampling infor"=w507, "Handle"=w512) -> ("error out"=w509:errorcluster, "Times&Values"=w508:T13, "handle"=w510:i16)  [unwired: 5 in]
        n187 = call "ps2000 Data Convert.vi"("Sampling infor"=w507, "pico Cluster"=w497, "Times&Values"=w508) -> ("wveform"=w486:waveform(dbl)[])  [unwired: 7 in, 1 out]
        n188 = Enqueue Element(queue=w504, element="read UI", error in (no error)=w506) -> (queue out=w503:refnum<queue>, error out=w505:errorcluster)  [unwired: 1 in, 1 out]
        n189 = case shown="\"5 V\"" w501 {
          tunnel: [0.011 0.021 0.051 0.11 0.21 0.51 1.1 2.1 5.1 10.1 20.1] -> w495
          frame "10 mV", Default {
          }
          frame "20 mV" {
          }
          frame "50 mV" {
          }
          frame "100 mV" {
          }
          frame "200 mV" {
          }
          frame "500 mV" {
          }
          frame "1 V" {
          }
          frame "2 V" {
          }
          frame "5 V" {
          }
          frame "10 V" {
          }
          frame "20 V" {
          }
        }
        n190 = case shown="\"1 V\"" w496 {
          tunnel: [0.011 0.021 0.051 0.11 0.21 0.51 1.1 2.1 5.1 10.1 20.1] -> w491
          frame "10 mV", Default {
          }
          frame "20 mV" {
          }
          frame "50 mV" {
          }
          frame "100 mV" {
          }
          frame "200 mV" {
          }
          frame "500 mV" {
          }
          frame "1 V" {
          }
          frame "2 V" {
          }
          frame "5 V" {
          }
          frame "10 V" {
          }
          frame "20 V" {
          }
        }
        n191 = Not(x="Play Button") -> (.not. x?=w488:bool)
        n192 = feedback #3() -> (w485:waveform(dbl)[])  [unwired: 1 in]
        n193 = Select(t=w486, s=w488, f=w485) -> (s? t:f=w484:waveform(dbl)[])
        n194 = feedback-in #3(w484) -> ()
        n195 = Multiply(x=w495, y=-1.0) -> (x*y=w494:dbl)
        n196 = Multiply(x=w491, y=-1.0) -> (x*y=w492:dbl)
        n197 = property on="Time" class="WFGraph (strict)"("ActYScl"=0 ("Active Y Scale"), "YScale.Maximum"=w495, "YScale.Minimum"=w494) -> ()  [unwired: 2 in, 2 out]
        n198 = property on="Time" class="WFGraph (strict)"("ActYScl"=1 ("Active Y Scale"), "YScale.Maximum"=w491, "YScale.Minimum"=w492) -> ()  [unwired: 2 in, 2 out]
        n199 = call "FFT 2 chan (SubVI).vi"("wveform"=w484) -> ("Array"=→"Freq":waveform(dbl)[])  [unwired: 9 in, 1 out]
        n200 = call "Offset 2 chan (SubVI).vi"("wveform"=w484, "pico Cluster"=w497) -> ("Waveform Graph"=→"Time":waveform(dbl)[])  [unwired: 8 in, 1 out]
      }
      frame "close" {
        n201 = call "ps2000 Close (SubVI).vi"("error in (no error)"=w543, "handle"=w541) -> ("error out"=w542:errorcluster)  [unwired: 8 in, 1 out]
      }
      frame "Idle", Default {
      }
    }
    n202 = case shown="Error" w355 {
      tunnel: w354 -> [w370 w376]
      tunnel: w353 -> [w369 w377]
      tunnel: [w370 w375] -> w352
      tunnel: [w369 w371] -> w351
      tunnel: w350 -> [_ w373]
      frame No Error {
      }
      frame Error {
        n203 = Enqueue Element At Opposite End(queue=w376, element="Close", error in (no error)=w377) -> (queue out=w375:refnum<queue>, error out=w372:errorcluster)  [unwired: 1 in, 1 out]
        n204 = call "TrapError (SubVI).vi"("error in (no error)"=w372, "stopEvent in"=w373) -> ("error out"=w371:errorcluster)  [unwired: 8 in, 1 out]
      }
    }
  }
  n205 = Release Notifier(notifier=w15, error in (no error)=w14) -> (error out=w13:errorcluster)  [unwired: 1 in, 2 out]
  n206 = Unregister For Events(event registration refnum=w29, error in=w13) -> (error out=w28:errorcluster)
  n207 = Destroy User Event(user event=w24, error in=w28) -> (error out=w27:errorcluster)
  n208 = Release Queue(queue=w4, error in (no error)=w3) -> (error out=w23:errorcluster)  [unwired: 1 in, 2 out]
  n209 = Merge Errors(w27, w25, w22, w23) -> (w26:errorcluster)
  n210 = call <vilib>:"Simple Error Handler.vi"("error in (no error)"=w26) -> ("error out"=w21:errorcluster)  [unwired: 4 in, 4 out]
  n211 = flat-sequence {
    tunnel: w21 -> [w551]
    tunnel: [w551] -> w20
    frame #0 {
      n212 = local write "stop"(FALSE ("stop")) -> ()
      n213 = property on="Cæng kÕt nèi" class="VISAName"("DisabledEnum"=T8."Enabled" ("Disabled")) -> ()  [unwired: 2 in, 2 out]
    }
  }
  n214 = disable-structure shown="RUN_TIME_ENGINE==True" {
    disable-tunnel: w20 -> [_ _]
    frame condition #0 (active) {
    }
    frame condition #1 {
      n215 = Quit LabVIEW(quit? (T)=TRUE) -> ()
    }
  }
